vi "WPI_CameraGet Image Sensor Property.vi"(8 "error in (no error)":errorcluster, 10 "Prop String":string, 11 "address":string="192.168.0.90") -> (0 "error out":errorcluster, 3 "Value":string)   [LabVIEW 2017]
doc: "This software is licensed. Open the labview\\readme\\WPI Robotics Library Open Source License.txt file for more information."
panel:
  out "Complete Response":string
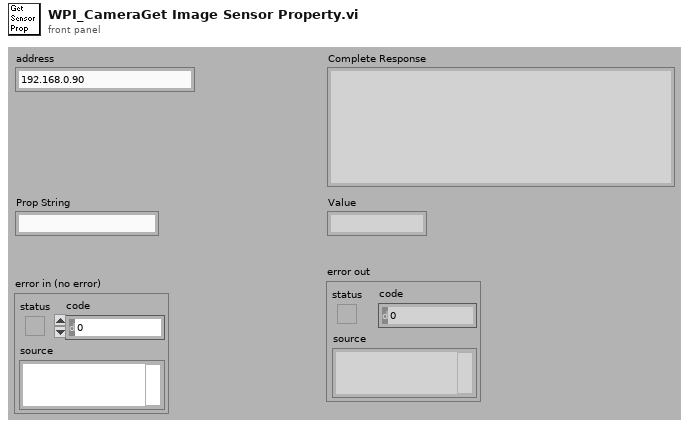
[diagram p1: front panel]
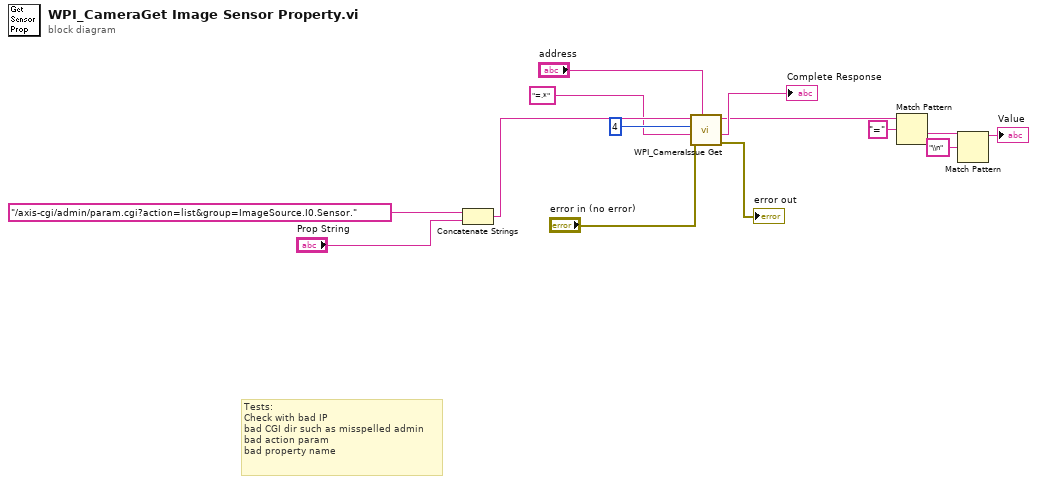
[diagram p0: block diagram]
diagram:
  # "Tests:\nCheck with bad IP\nbad CGI dir such as misspelled admin\nbad action param\nbad property name"
  n1 = Concatenate Strings("/axis-cgi/admin/param.cgi?action=list&group=ImageSource.I0.Sensor.", "Prop String") -> (w11:string)
  n2 = call <vilib>:"WPI_CameraIssue Get.vi"("address"="address", "error in (no error)"="error in (no error)", "Regular Expression of text to extract"="=.*", "Number of Lines Expected"=4, "Request"=w11) -> ("error out"=→"error out":errorcluster, "Complete Response"=→"Complete Response":string, "Extracted String"=w7:string)  [unwired: 4 out]
  n3 = Match Pattern(string=w7, regular expression="=") -> (after substring=w5:string)  [unwired: 4 out]
  n4 = Match Pattern(string=w5, regular expression="\\n") -> (before substring=→"Value":string)  [unwired: 4 out]
